vi "Write Cooker.vi"(8 "error in (no error)":errorcluster, 10 "Cooker Message Enqueuer":refnum<class "Message Enqueuer.lvclass">, 11 "Chef State in":refnum<class "Chef State.lvclass">) -> (0 "error out":errorcluster, 3 "Chef State out":refnum<class "Chef State.lvclass">)   [LabVIEW 2024, in "Chef States.lvlib" / "Chef State.lvclass"]
uses:
  Chef State.lvclass
  <vilib>/ActorFramework/Message Enqueuer/Message Enqueuer.lvclass
  Chef State.lvclass/Chef State.ctl
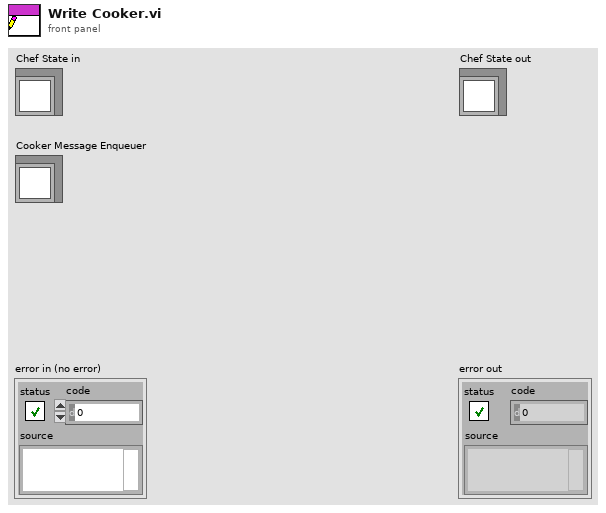
[diagram p1: front panel]
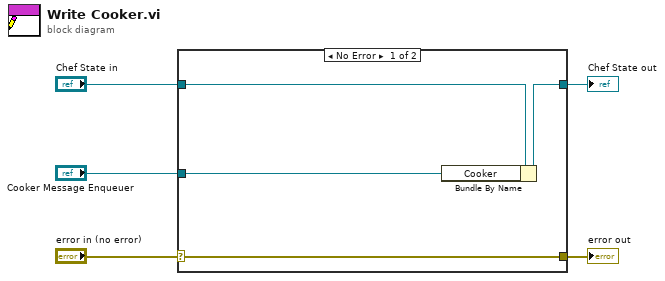
[diagram p0: block diagram]
diagram:
  n1 = case shown="No Error" "error in (no error)" {
    selector: "error in (no error)" -> [w9 w10]
    tunnel: [w9 w10] -> w4
    tunnel: [w7 w11] -> w2
    tunnel: "Chef State in" -> [w8 w11]
    tunnel: "Cooker Message Enqueuer" -> [w6 _]
    frame No Error {
      n2 = Bundle By Name(cluster=w8, "Cooker"=w6) -> (w7:refnum<class "Chef State.lvclass">)
    }
    frame Error {
    }
  }
  "error out" <- w4
  "Chef State out" <- w2
